vi "State_Machine.vi"(8 "error in (no error)":errorcluster caption="entrée d'erreur (pas d'erreur)", 11 "Get_Voltage en entrée":refnum<class "Zigbee_Write_Msg.lvclass">) -> (0 "error out":errorcluster caption="sortie d'erreur", 2 "Json_String":string, 3 "Get_Voltage en sortie":refnum<class "Zigbee_Write_Msg.lvclass">)   [LabVIEW 2020, in "Library Test.lvlib" / "Zigbee_Write_Msg.lvclass"]
uses:
  Zigbee_Write_Msg.lvclass
  C:/Users/ngarcin/OneDrive - Altyor/Standard TB/Class/Test/Test (Default)/Test (Default).lvclass
  C:/Users/ngarcin/OneDrive - Altyor/Standard TB/Class/Test/Zigbee_Send_Command_UART/Zigbee_Send_Command_UART.lvclass
  JSON API/JSON Value/Set from JSON string.vi
  JSON API/JSON Value/JSON Value.lvclass
  Zigbee_Send_Command_UART/Zigbee_Send_Command_UART.lvclass
  Zigbee_Write_Msg.lvclass/Zigbee_Write_Msg.ctl
  JSON API/Variant JSON/Variant JSON.lvlib
  JSON API/Get Polymorphic/JSON GetSet.lvlib
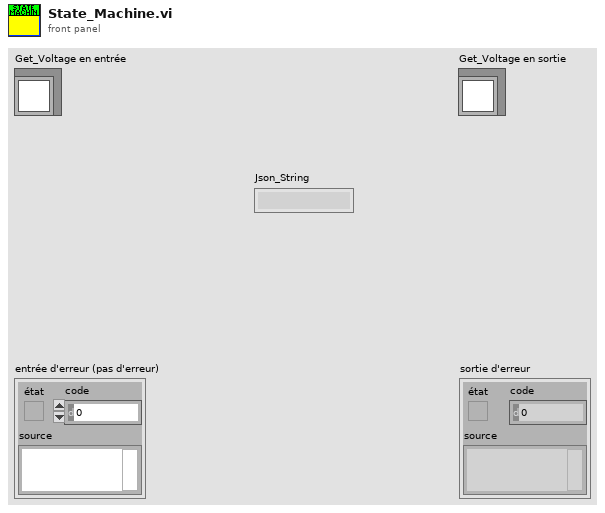
[diagram p1: front panel]
types:
  T1 = cluster{"Cluster":string, "attributeId":string, "Data":string, "TypeData":string}
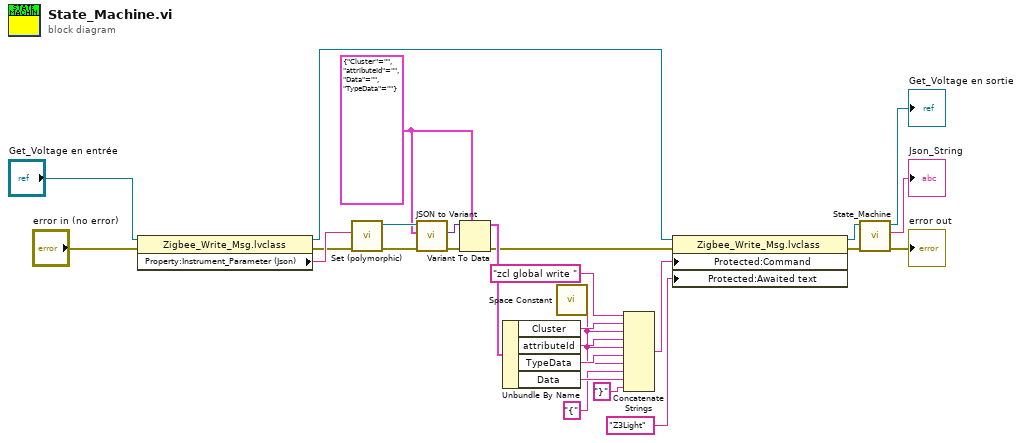
[diagram p0: block diagram]
diagram:
  w16 = T1 {"Cluster"="", "attributeId"="", "Data"="", "TypeData"=""}
  n1 = property class="Zigbee_Write_Msg.lvclass"(reference="Get_Voltage en entrée", error in="error in (no error)") -> (reference out=w12:refnum<class "Zigbee_Write_Msg.lvclass">, error out=w17:errorcluster, "Property:Instrument_Parameter (Json)"=w18:string)
  n2 = call-poly "Set (polymorphic).vi"("error in (no error)"=w17, "JSON stream"=w18) -> ("error out"=w20:errorcluster, "JSON Value out"=w22:refnum<class "JSON Value.lvclass">)  [unwired: 7 in, 1 out]
  n3 = call "JSON to Variant.vi"("error in (no error)"=w20, "Variant (Data Type)"=w16, "JSON Value"=w22) -> ("error out"=w21:errorcluster, "Variant out"=w19:variant)  [unwired: 7 in]
  n4 = Variant To Data(error in=w21, type=w16, Variant=w19) -> (data=w15:T1, error out=w11:errorcluster)
  n5 = Unbundle By Name(w15) -> ("Cluster"=w8:string, "attributeId"=w7:string, "TypeData"=w2:string, "Data"=w6:string)
  n6 = call <vilib>:"Space Constant.vi"() -> ("String"=w1:string)
  n7 = Concatenate Strings("zcl global write " ("Command"), w8, w1, w7, w1, w2, w1, "{" ("chaîne"), w6, "}" ("chaîne")) -> (w9:string)
  n8 = property class="Zigbee_Write_Msg.lvclass"(reference=w12, error in=w11, "Protected:Command"=w9, "Protected:Awaited text"="Z3Light" ("Awaited text")) -> (reference out=w24:refnum<class "Zigbee_Write_Msg.lvclass">, error out=w23:errorcluster)
  n9 = call-parent "State_Machine.vi"("error in (no error)"=w23, "Send_Frame en entrée"=w24) -> ("error out"=→"error out":errorcluster, "Json_String"=→"Json_String":string, "Send_Frame en sortie"=→"Get_Voltage en sortie":refnum<class "Zigbee_Write_Msg.lvclass">)  [unwired: 7 in]
